vi "回文数与水仙花数判断(上).vi"() -> ()   [LabVIEW 2018]
panel:
  out "s? t:f":string
  out "回文数判断：":string
  out "?":bool
  in  "数值":i64
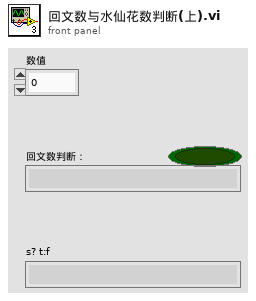
[diagram p1: front panel]
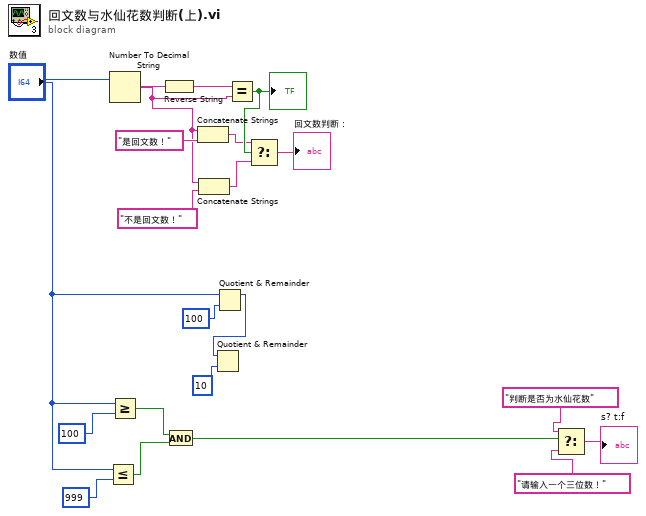
[diagram p0: block diagram]
diagram:
  n1 = Less Or Equal?(x="数值", y=999) -> (x <= y?=w10:bool)
  n2 = Number To Decimal String(number="数值") -> (decimal integer string=w15:string)  [unwired: 1 in]
  n3 = Greater Or Equal?(x="数值", y=100) -> (x >= y?=w9:bool)
  n4 = Reverse String(1:w15) -> (0:w20:string)
  n5 = And(x=w9, y=w10) -> (x .and. y?=w8:bool)
  n6 = Concatenate Strings(w15, "是回文数！") -> (w17:string)
  n7 = Concatenate Strings(w15, "不是回文数！") -> (w14:string)
  n8 = Quotient & Remainder(x="数值", y=100) -> (x-y*floor(x/y)=w1:i64)  [unwired: 1 out]
  n9 = Quotient & Remainder(x=w1, y=10) -> ()  [unwired: 2 out]
  n10 = Equal?(x=w20, y=w15) -> (x = y?=w19:bool)
  "?" <- w19
  n11 = Select(t=w17, s=w19, f=w14) -> (s? t:f=→"回文数判断：":string)
  n12 = Select(t="判断是否为水仙花数", s=w8, f="请输入一个三位数！") -> (s? t:f=→"s? t:f":string)
